vi "SmartPathToString.vi"(1 "output file":path) -> (0 "string":string)   [LabVIEW 2017, in "LabVIEWHTTPClient.lvlib"]
uses:
  LabVIEWHTTPClient.lvlib
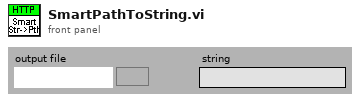
[diagram p1: front panel]
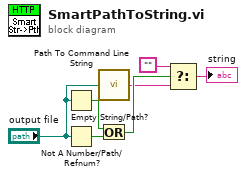
[diagram p0: block diagram]
diagram:
  n1 = Empty String/Path?(string/path="output file") -> (empty?=w5:bool)
  n2 = Not A Number/Path/Refnum?(number/path/refnum="output file") -> (NaN/Path/Refnum?=w4:bool)
  n3 = call "Path To Command Line String.vi"("path"="output file") -> ("string"=w1:string)
  n4 = Or(x=w5, y=w4) -> (x .or. y?=w3:bool)
  n5 = Select(t="", s=w3, f=w1) -> (s? t:f=→"string":string)
